vi "MultiSteps.vi"(0 "Connection Cluster in":T1, 1 "Coarse peak position":dbl) -> (14 "Connection Cluster out":T1, 16 "Peak position":dbl)   [LabVIEW 2013]
uses:
  Global.vi
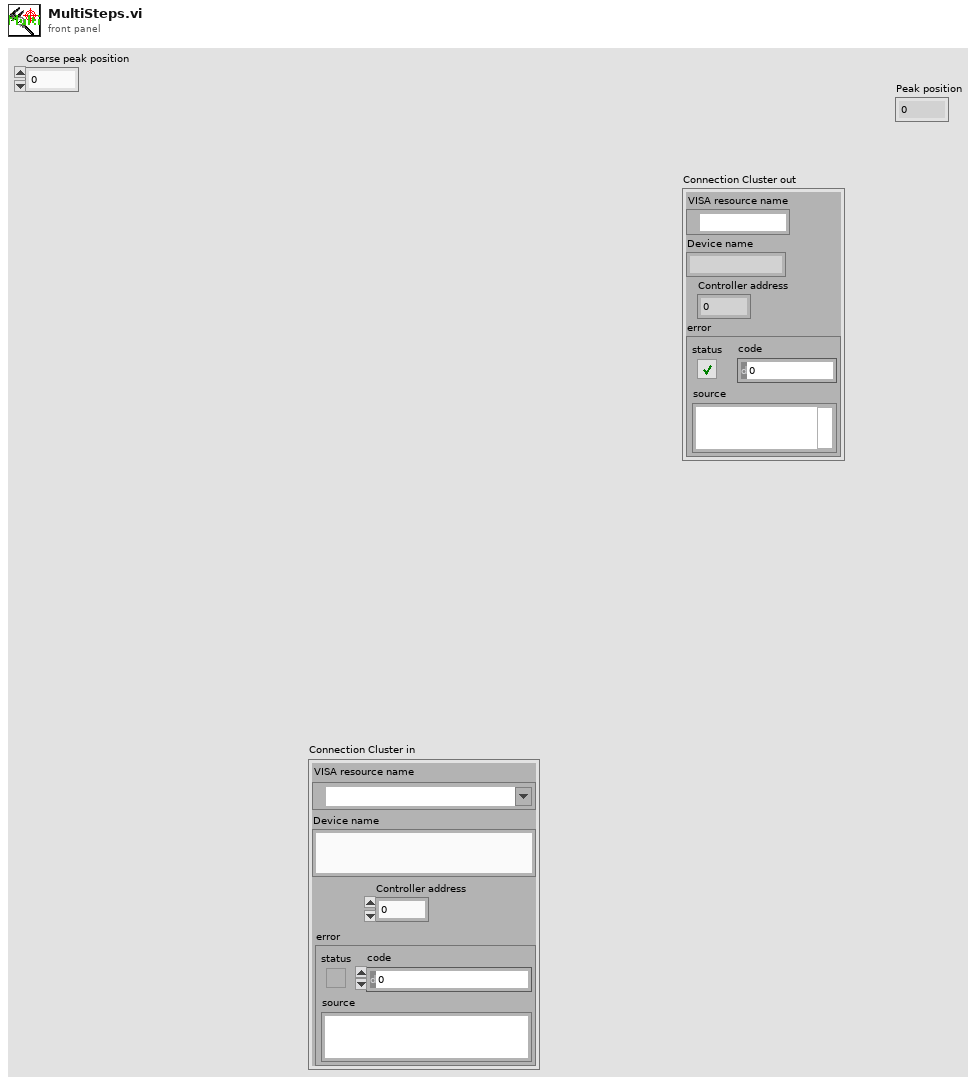
[diagram p1: front panel]
types:
  T1 = cluster{"VISA resource name":refnum<visa-resource-name>, "Device name":string, "Controller address":i32, "error":errorcluster}
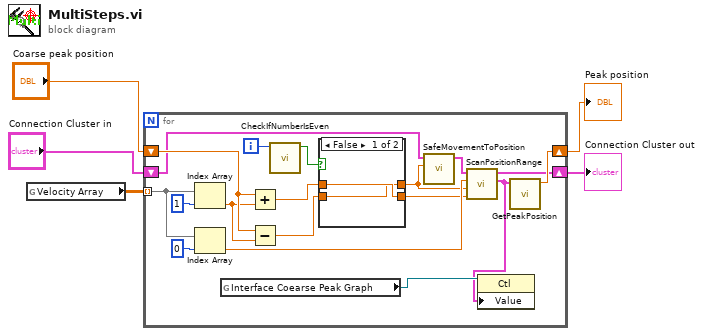
[diagram p0: block diagram]
diagram:
  n1 = global read "Global.vi" "Velocity Array"() -> (w5:dbl[][])
  n2 = for {
    tunnel: w5 -> [w22] mode=indexing
    shift-right: [w15] -> w4
    shift-left: "Connection Cluster in" -> [w16]
    shift-right: [w18] -> w3
    shift-left: "Coarse peak position" -> [w20]
    i -> [w17]
    n3 = Index Array(array=w22, index=1) -> (element=w19:dbl)
    n4 = Index Array(array=w22, index=0) -> (element=w14:dbl)
    n5 = global read "Global.vi" "Interface Coearse Peak Graph"() -> (w7:refnum<vi>)
    n6 = Add(x=w20, y=w19) -> (x+y=w11:dbl)
    n7 = Subtract(x=w20, y=w19) -> (x-y=w10:dbl)
    n8 = call "CheckIfNumberIsEven.vi"("x"=w17) -> ("even?"=w12:bool)  [unwired: 10 in]
    n9 = case shown="False" w12 {
      tunnel: w11 -> [w25 w27]
      tunnel: w10 -> [w24 w26]
      tunnel: [w24 w27] -> w9
      tunnel: [w25 w26] -> w8
      frame False {
      }
      frame True {
      }
    }
    n10 = call "SafeMovementToPosition.vi"("Target position"=w9, "Connection Cluster in"=w16) -> ("Connection Cluster out"=w13:T1)  [unwired: 9 in]
    n11 = call "ScanPositionRange.vi"("Target position"=w8, "Start position"=w9, "Velocity"=w14, "Connection Cluster in"=w13) -> ("output cluster"=w6:cluster{dbl[], dbl[]}, "Connection Cluster out"=w15:T1)  [unwired: 5 in, 1 out]
    n12 = property class="Ctl"(reference=w7, "Value"=w6) -> ()  [unwired: 1 in, 2 out]
    n13 = call "GetPeakPosition.vi"("Input cluster"=w6) -> ("Peak position [mm]"=w18:dbl)  [unwired: 10 in]
  }
  "Connection Cluster out" <- w4
  "Peak position" <- w3
